vi "ep_Flicker Level Classifier.vi"(0 "flicker cumulative probability function":dbl[](array[numeric])) -> (4 "flicker Pst":dbl)   [LabVIEW 2011, in "NI_EP_Power Quality.lvlib"]
uses:
  <vilib>/addons/Electrical Power/PQ/NI_EP_Power Quality.lvlib
panel:
  out "702 classes":dbl[](array[numeric])
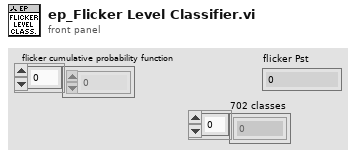
[diagram p1: front panel]
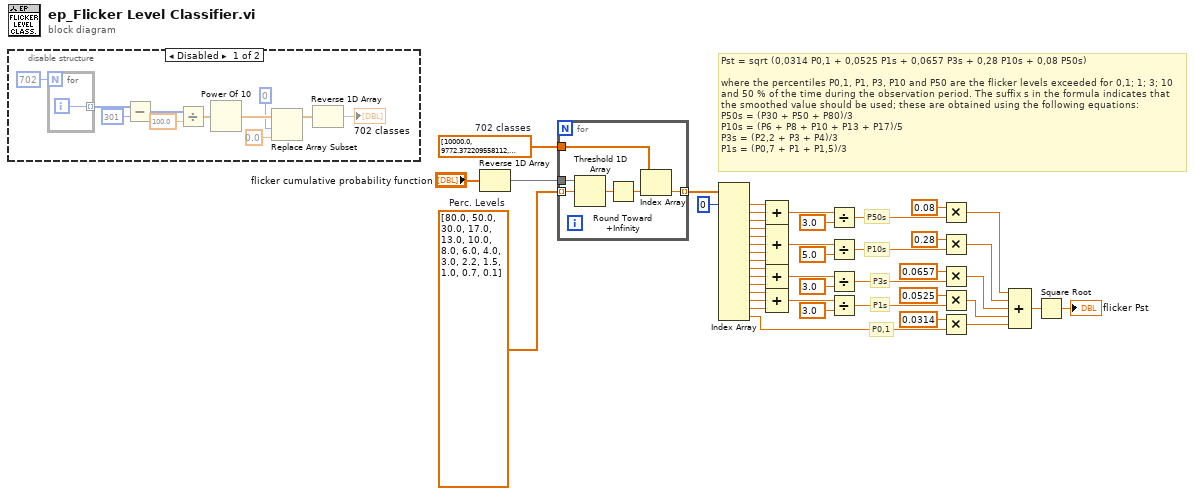
[diagram p0: block diagram]
diagram:
  w45 = dbl[] [10000.0, 9772.372209558112, 9549.92586021436, 9332.543007969914, 9120.108393559096, 8912.509381337459, 8709.635899560806, 8511.380382023768, 8317.63771102671, 8128.305161640995, 7943.282347242814, 7762.4711662869195, 7585.775750291836, 7413.102413009177, 7244.359600749898, 7079.457843841381, 6918.309709189362, 6760.829753919819, 6606.934480075957, 6456.542290346556, 6309.57344480193, 6165.9500186148225, 6025.595860743575, 5888.43655355589, 5754.399373371566, 5623.413251903491, 5495.408738576249, 5370.317963702527, 5248.074602497728, 5128.613839913648, 5011.872336272725, 4897.7881936844615, 4786.300923226385, 4677.351412871981, 4570.881896148751, 4466.835921509631, 4365.158322401661, 4265.795188015925, 4168.693834703355, 4073.802778041126, 3981.0717055349733, 3890.4514499428046, 3801.8939632056126, 3715.352290971724, 3630.780547701014, 3548.133892335753, 3467.368504525317, 3388.441561392024, 3311.311214825911, 3235.936569296281, 3162.2776601683795, 3090.295432513592, 3019.9517204020162, 2951.209226666387, 2884.031503126606, 2818.382931264455, 2754.2287033381663, 2691.5348039269165, 2630.2679918953813, 2570.3957827688646, 2511.88643150958, 2454.708915685031, 2398.83291901949, 2344.228815319923, 2290.8676527677726, 2238.72113856834, 2187.761623949552, 2137.9620895022326, 2089.296130854039, 2041.7379446695295, 1995.2623149688789, 1949.8445997580454, 1905.4607179632462, 1862.0871366628676, 1819.7008586099826, 1778.2794100389228, 1737.8008287493763, 1698.2436524617442, 1659.5869074375614, 1621.8100973589299, 1584.893192461114, 1548.816618912481, 1513.5612484362086, 1479.1083881682073, 1445.439770745928, 1412.537544622754, 1380.3842646028852, 1348.9628825916532, 1318.2567385564075, 1288.2495516931335, 1258.9254117941675, 1230.268770812381, 1202.2644346174131, 1174.897554939529, 1148.1536214968828, 1122.018454301963, 1096.4781961431852, 1071.519305237606, 1047.1285480508996, 1023.2929922807537, 1000.0, 977.2372209558112, 954.992586021436, 933.2543007969915, 912.0108393559096, 891.2509381337459, 870.9635899560806, 851.1380382023768, 831.7637711026708, 812.8305161640995, 794.3282347242813, 776.247116628692, 758.5775750291835, 741.3102413009177, 724.4359600749899, 707.945784384138, 691.8309709189363, 676.0829753919819, 660.6934480075957, 645.6542290346556, 630.957344480193, 616.5950018614822, 602.5595860743575, 588.843655355589, 575.4399373371566, 562.341325190349, 549.5408738576248, 537.0317963702527, 524.8074602497728, 512.8613839913648, 501.18723362727246, 489.77881936844614, 478.6300923226385, 467.73514128719813, 457.0881896148752, 446.683592150963, 436.5158322401661, 426.57951880159254, 416.8693834703355, 407.3802778041126, 398.1071705534973, 389.04514499428046, 380.1893963205613, 371.5352290971724, 363.0780547701014, 354.8133892335753, 346.73685045253166, 338.84415613920237, 331.1311214825911, 323.5936569296281, 316.22776601683796, 309.0295432513592, 301.9951720402016, 295.1209226666387, 288.40315031266056, 281.8382931264455, 275.4228703338166, 269.1534803926917, 263.02679918953817, 257.03957827688646, 251.18864315095797, 245.4708915685031, 239.88329190194898, 234.42288153199226, 229.08676527677724, 223.872113856834, 218.77616239495518, 213.79620895022325, 208.92961308540387, 204.17379446695296, 199.52623149688787, 194.98445997580455, 190.54607179632464, 186.20871366628674, 181.97008586099827, 177.82794100389228, 173.78008287493762, 169.82436524617444, 165.95869074375614, 162.18100973589299, 158.48931924611142, 154.88166189124811, 151.35612484362088, 147.91083881682073, 144.5439770745928, 141.2537544622754, 138.03842646028852, 134.89628825916532, 131.82567385564073, 128.82495516931337, 125.89254117941675, 123.02687708123811, 120.22644346174131, 117.48975549395291, 114.81536214968828, 112.2018454301963, 109.64781961431851, 107.1519305237606, 104.71285480508996, 102.32929922807536, 100.0, 97.72372209558107, 95.49925860214358, 93.3254300796991, 91.20108393559097, 89.12509381337455, 87.09635899560806, 85.11380382023764, 83.17637711026708, 81.2830516164099, 79.43282347242814, 77.62471166286916, 75.85775750291836, 74.13102413009177, 72.44359600749902, 70.79457843841381, 69.18309709189366, 67.60829753919819, 66.06934480075961, 64.56542290346556, 63.09573444801933, 61.65950018614822, 60.25595860743578, 58.8843655355589, 57.543993733715695, 56.23413251903491, 54.954087385762456, 53.70317963702527, 52.48074602497726, 51.28613839913648, 50.11872336272722, 48.97788193684461, 47.86300923226383, 46.77351412871981, 45.708818961487495, 44.6683592150963, 43.65158322401658, 42.65795188015925, 41.68693834703355, 40.73802778041128, 39.810717055349734, 38.90451449942807, 38.018939632056124, 37.15352290971726, 36.30780547701014, 35.48133892335755, 34.673685045253166, 33.884415613920254, 33.11311214825911, 32.359365692962825, 31.622776601683793, 30.902954325135905, 30.19951720402016, 29.512092266663856, 28.84031503126606, 28.183829312644534, 27.542287033381662, 26.915348039269155, 26.302679918953814, 25.703957827688633, 25.118864315095795, 24.547089156850298, 23.9883291901949, 23.442288153199225, 22.908676527677734, 22.3872113856834, 21.87761623949553, 21.379620895022324, 20.892961308540396, 20.417379446695296, 19.952623149688797, 19.498445997580454, 19.054607179632473, 18.620871366628677, 18.197008586099834, 17.78279410038923, 17.378008287493753, 16.982436524617444, 16.595869074375607, 16.218100973589298, 15.848931924611133, 15.488166189124811, 15.13561248436208, 14.791083881682072, 14.454397707459272, 14.12537544622754, 13.803842646028846, 13.489628825916533, 13.182567385564074, 12.882495516931343, 12.589254117941675, 12.302687708123818, 12.02264434617413, 11.748975549395297, 11.481536214968829, 11.220184543019636, 10.964781961431852, 10.715193052376065, 10.471285480508996, 10.232929922807541, 10.0, 9.772372209558107, 9.549925860214358, 9.33254300796991, 9.120108393559097, 8.912509381337454, 8.709635899560805, 8.511380382023766, 8.31763771102671, 8.128305161640993, 7.943282347242816, 7.762471166286917, 7.5857757502918375, 7.413102413009175, 7.244359600749901, 7.079457843841379, 6.918309709189364, 6.760829753919817, 6.606934480075959, 6.456542290346556, 6.309573444801933, 6.165950018614822, 6.025595860743578, 5.88843655355589, 5.7543993733715695, 5.623413251903491, 5.495408738576246, 5.370317963702527, 5.248074602497725, 5.1286138399136485, 5.011872336272722, 4.897788193684462, 4.786300923226384, 4.677351412871983, 4.570881896148751, 4.466835921509632, 4.36515832240166, 4.265795188015927, 4.168693834703354, 4.073802778041127, 3.9810717055349722, 3.890451449942806, 3.8018939632056115, 3.715352290971725, 3.630780547701014, 3.548133892335755, 3.4673685045253166, 3.3884415613920256, 3.311311214825911, 3.2359365692962827, 3.1622776601683795, 3.0902954325135905, 3.019951720402016, 2.9512092266663856, 2.884031503126606, 2.8183829312644537, 2.7542287033381663, 2.6915348039269156, 2.6302679918953817, 2.5703957827688635, 2.51188643150958, 2.4547089156850306, 2.3988329190194904, 2.344228815319922, 2.290867652767773, 2.2387211385683394, 2.1877616239495525, 2.137962089502232, 2.0892961308540396, 2.041737944669529, 1.9952623149688795, 1.9498445997580451, 1.9054607179632472, 1.8620871366628675, 1.8197008586099834, 1.7782794100389228, 1.7378008287493754, 1.6982436524617444, 1.6595869074375607, 1.62181009735893, 1.5848931924611136, 1.5488166189124815, 1.5135612484362082, 1.4791083881682074, 1.4454397707459274, 1.4125375446227544, 1.3803842646028848, 1.3489628825916535, 1.318256738556407, 1.288249551693134, 1.2589254117941673, 1.2302687708123816, 1.202264434617413, 1.1748975549395295, 1.1481536214968828, 1.1220184543019633, 1.096478196143185, 1.0715193052376064, 1.0471285480508996, 1.023292992280754, 1.0, 0.9772372209558107, 0.954992586021436, 0.933254300796991, 0.9120108393559098, 0.8912509381337456, 0.8709635899560807, 0.8511380382023764, 0.831763771102671, 0.8128305161640993, 0.7943282347242815, 0.7762471166286917, 0.7585775750291838, 0.7413102413009175, 0.72443596007499, 0.7079457843841379, 0.6918309709189365, 0.6760829753919817, 0.660693448007596, 0.6456542290346555, 0.6309573444801932, 0.6165950018614822, 0.6025595860743578, 0.5888436553555889, 0.5754399373371569, 0.5623413251903491, 0.5495408738576245, 0.5370317963702527, 0.5248074602497725, 0.5128613839913648, 0.5011872336272722, 0.4897788193684462, 0.4786300923226383, 0.4677351412871982, 0.457088189614875, 0.44668359215096315, 0.436515832240166, 0.42657951880159267, 0.4168693834703354, 0.40738027780411273, 0.3981071705534972, 0.3890451449942806, 0.3801893963205612, 0.37153522909717257, 0.36307805477010135, 0.35481338923357547, 0.3467368504525316, 0.33884415613920255, 0.3311311214825911, 0.32359365692962827, 0.31622776601683794, 0.30902954325135906, 0.3019951720402016, 0.29512092266663853, 0.28840315031266056, 0.28183829312644537, 0.2754228703338166, 0.2691534803926916, 0.2630267991895382, 0.2570395782768864, 0.251188643150958, 0.24547089156850305, 0.23988329190194904, 0.2344228815319922, 0.2290867652767773, 0.22387211385683395, 0.21877616239495523, 0.2137962089502232, 0.20892961308540392, 0.20417379446695297, 0.19952623149688797, 0.19498445997580455, 0.19054607179632474, 0.18620871366628675, 0.18197008586099836, 0.1778279410038923, 0.17378008287493754, 0.16982436524617442, 0.16595869074375605, 0.16218100973589297, 0.15848931924611134, 0.1548816618912481, 0.15135612484362082, 0.14791083881682077, 0.14454397707459277, 0.14125375446227545, 0.1380384264602885, 0.13489628825916536, 0.1318256738556407, 0.1288249551693134, 0.12589254117941673, 0.12302687708123815, 0.12022644346174129, 0.11748975549395294, 0.1148153621496883, 0.11220184543019636, 0.1096478196143185, 0.10715193052376065, 0.10471285480508996, 0.10232929922807542, 0.1, 0.09772372209558107, 0.09549925860214359, 0.0933254300796991, 0.09120108393559097, 0.08912509381337455, 0.08709635899560805, 0.08511380382023763, 0.08317637711026708, 0.0812830516164099, 0.07943282347242814, 0.07762471166286916, 0.07585775750291836, 0.07413102413009177, 0.07244359600749903, 0.0707945784384138, 0.06918309709189366, 0.06760829753919818, 0.06606934480075961, 0.06456542290346556, 0.06309573444801933, 0.06165950018614822, 0.06025595860743578, 0.0588843655355589, 0.057543993733715694, 0.05623413251903491, 0.054954087385762455, 0.05370317963702527, 0.05248074602497726, 0.05128613839913648, 0.05011872336272722, 0.04897788193684462, 0.047863009232263824, 0.046773514128719815, 0.04570881896148749, 0.0446683592150963, 0.043651583224016584, 0.04265795188015926, 0.04168693834703355, 0.04073802778041128, 0.039810717055349734, 0.03890451449942807, 0.038018939632056124, 0.03715352290971726, 0.03630780547701014, 0.03548133892335755, 0.034673685045253165, 0.033884415613920256, 0.03311311214825911, 0.03235936569296283, 0.03162277660168379, 0.030902954325135904, 0.03019951720402016, 0.029512092266663854, 0.028840315031266057, 0.028183829312644536, 0.02754228703338166, 0.026915348039269153, 0.026302679918953815, 0.025703957827688632, 0.025118864315095794, 0.024547089156850298, 0.023988329190194897, 0.023442288153199226, 0.022908676527677734, 0.0223872113856834, 0.02187761623949553, 0.021379620895022326, 0.020892961308540396, 0.020417379446695295, 0.0199526231496888, 0.019498445997580455, 0.019054607179632473, 0.018620871366628676, 0.018197008586099836, 0.01778279410038923, 0.017378008287493755, 0.016982436524617443, 0.016595869074375606, 0.0162181009735893, 0.015848931924611134, 0.01548816618912481, 0.01513561248436208, 0.014791083881682071, 0.014454397707459272, 0.01412537544622754, 0.013803842646028845, 0.013489628825916533, 0.013182567385564075, 0.012882495516931342, 0.012589254117941675, 0.012302687708123818, 0.012022644346174132, 0.011748975549395297, 0.01148153621496883, 0.011220184543019636, 0.01096478196143185, 0.010715193052376065, 0.010471285480508996, 0.010232929922807542, 0.01, 0.009772372209558112, 0.009549925860214359, 0.009332543007969915, 0.009120108393559097, 0.008912509381337459, 0.008709635899560805, 0.008511380382023767, 0.008317637711026709, 0.008128305161640995, 0.007943282347242814, 0.00776247116628692, 0.007585775750291836, 0.007413102413009177, 0.007244359600749898, 0.00707945784384138, 0.006918309709189363, 0.006760829753919818, 0.006606934480075957, 0.006456542290346556, 0.00630957344480193, 0.006165950018614822, 0.006025595860743574, 0.00588843655355589, 0.005754399373371567, 0.005623413251903491, 0.005495408738576248, 0.005370317963702527, 0.005248074602497728, 0.005128613839913648, 0.005011872336272725, 0.004897788193684461, 0.004786300923226385, 0.004677351412871981, 0.004570881896148752, 0.0044668359215096305, 0.004365158322401661, 0.004265795188015926, 0.004168693834703355, 0.004073802778041126, 0.003981071705534973, 0.003890451449942805, 0.0038018939632056127, 0.003715352290971724, 0.003630780547701014, 0.0035481338923357532, 0.0034673685045253167, 0.003388441561392024, 0.003311311214825911, 0.003235936569296281, 0.0031622776601683794, 0.003090295432513592, 0.003019951720402016, 0.002951209226666387, 0.002884031503126606, 0.002818382931264455, 0.002754228703338166, 0.0026915348039269166, 0.0026302679918953813, 0.0025703957827688645, 0.0025118864315095794, 0.002454708915685031, 0.00239883291901949, 0.0023442288153199225, 0.0022908676527677724, 0.00223872113856834, 0.002187761623949552, 0.0021379620895022326, 0.0020892961308540386, 0.0020417379446695297, 0.001995262314968879, 0.0019498445997580456, 0.0019054607179632462, 0.0018620871366628676, 0.0018197008586099826, 0.0017782794100389228, 0.0017378008287493763, 0.0016982436524617442, 0.0016595869074375613, 0.0016218100973589297, 0.001584893192461114, 0.0015488166189124811, 0.0015135612484362087, 0.0014791083881682072, 0.001445439770745928, 0.001412537544622754, 0.0013803842646028853, 0.0013489628825916532, 0.0013182567385564075, 0.0012882495516931337, 0.0012589254117941675, 0.0012302687708123812, 0.001202264434617413, 0.001174897554939529, 0.0011481536214968829, 0.001122018454301963, 0.0010964781961431851, 0.001071519305237606, 0.0010471285480508996, 0.0010232929922807535, 0.001, 0.0]  # 702 classes
  w42 = dbl[] [80.0, 50.0, 30.0, 17.0, 13.0, 10.0, 8.0, 6.0, 4.0, 3.0, 2.2, 1.5, 1.0, 0.7, 0.1]  # Perc. Levels
  # "Pst = sqrt (0,0314 P0,1 + 0,0525 P1s + 0,0657 P3s + 0,28 P10s + 0,08 P50s)\n\nwhere the percentiles P0,1, P1, P3, P10 and P50 are the flicker levels exceeded for 0,1; 1; 3; 10\nand 50 % of the time during the observation period. The suffix s in the formula indicates that\nthe smoothed value should be used; these are obtained using the following equations:\nP50s = (P30 + P50 + P80)/3\nP10s = (P6 + P8 + P10 + P13 + P17)/5\nP3s = (P2,2 + P3 + P4)/3\nP1s = (P0,7 + P1 + P1,5)/3"
  # "P10s"
  # "P0,1"
  # "P1s"
  # "P3s"
  # "P50s"
  n1 = disable-structure shown="Disabled" {
    frame Disabled {
      n2 = for {
        N: 702 -> [_]
        tunnel: [w57] -> w51 mode=indexing
        i -> [w57]
      }
      n3 = Subtract(x=w51, y=301) -> (x-y=w55:i32[])
      n4 = Divide(x=w55, y=100.0) -> (x/y=w54:dbl[])
      n5 = Power Of 10(x=w54) -> (10^x=w50:dbl[])
      n6 = Replace Array Subset(array=w50, new element=0.0 ("new element/subarray"), index=0) -> (w49:dbl[])
      n7 = Reverse 1D Array(array=w49) -> (reversed array=→"702 classes":dbl[])
    }
    frame Enabled {
    }
  }
  n8 = Reverse 1D Array(array="flicker cumulative probability function") -> (reversed array=w43:dbl[])
  n9 = for {
    tunnel: w42 -> [w62] mode=indexing
    tunnel: w43 -> [w63]
    tunnel: w45 -> [w61]
    tunnel: [w60] -> w44 mode=indexing
    n10 = Threshold 1D Array(2:w62, 3:w63) -> (0:w59:dbl)  [unwired: 1 in]
    n11 = Round Toward +Infinity(x=w59) -> (ceil(x): smallest int >= x=w58:dbl)
    n12 = Index Array(array=w61, index=w58) -> (element=w60:dbl)
  }
  n13 = Index Array(array=w44, index #1=0 ("index")) -> (element #1=w34:dbl, element #2=w35:dbl, element #3=w36:dbl, element #4=w13:dbl, element #5=w15:dbl, element #6=w16:dbl, element #7=w17:dbl, element #8=w18:dbl, element #9=w25:dbl, element #10=w26:dbl, element #11=w27:dbl, element #12=w29:dbl, element #13=w30:dbl, element #14=w31:dbl, element #15=w33:dbl)  [unwired: 14 in]
  n14 = Compound Arithmetic op=ADD(w34, w35, w36) -> (w38:dbl)
  n15 = Compound Arithmetic op=ADD(w13, w15, w16, w17, w18) -> (w14:dbl)
  n16 = Compound Arithmetic op=ADD(w25, w26, w27) -> (w28:dbl)
  n17 = Compound Arithmetic op=ADD(w29, w30, w31) -> (w32:dbl)
  n18 = Divide(x=w38, y=3.0) -> (x/y=w39:dbl)
  n19 = Divide(x=w14, y=5.0) -> (x/y=w9:dbl)
  n20 = Divide(x=w28, y=3.0) -> (x/y=w10:dbl)
  n21 = Divide(x=w32, y=3.0) -> (x/y=w11:dbl)
  n22 = Multiply(x=0.08, y=w39) -> (x*y=w19:dbl)
  n23 = Multiply(x=0.28, y=w9) -> (x*y=w20:dbl)
  n24 = Multiply(x=0.0657, y=w10) -> (x*y=w21:dbl)
  n25 = Multiply(x=0.0525, y=w11) -> (x*y=w22:dbl)
  n26 = Multiply(x=0.0314, y=w33) -> (x*y=w23:dbl)
  n27 = Compound Arithmetic op=ADD(w19, w20, w21, w22, w23) -> (w24:dbl)
  n28 = Square Root(x=w24) -> (sqrt(x)=→"flicker Pst":dbl)
